vi "Unlock Data.vi"(8 "error in (no error)":errorcluster, 9 "Datum Type":variant, 10 "Datum Name":string, 11 "IModel in":refnum<class "IModel.lvclass">) -> (0 "error out":errorcluster, 3 "IModel out":refnum<class "IModel.lvclass">)   [LabVIEW 2015, in "IModel.lvlib" / "IModel.lvclass"]
doc: "Publish a datum (value) to the mediator bus. Published data are observable by any actor with access to the mediated bus."
uses:
  IModel.lvclass
  <vilib>/ActorFramework/Actor/Actor.lvclass/Actor.ctl
  <vilib>/ActorFramework/Message Enqueuer/Message Enqueuer.lvclass/Message Enqueuer.ctl
  IModel.lvclass/IModel.ctl
  AbstractMessages/PreAddressedMsg/PreAddressedMsg.lvclass/PreAddressedMsg.ctl
  IMediator/IMediator Messages/Unlock Publication Msg/Unlock Publication Msg.lvclass/Unlock Publication Msg.ctl
  <vilib>/ActorFramework/Actor/Read Self Enqueuer.vi
  <vilib>/ActorFramework/Message Enqueuer/Enqueue.vi
  AbstractMessages/PreAddressedMsg/Read Return Address.vi
  <vilib>/ActorFramework/Message Enqueuer/Init from Existing Queue.vi
  <vilib>/ActorFramework/Message Priority Queue/Priority Enqueue.vi
  <vilib>/ActorFramework/Message Enqueuer/Message Enqueuer.lvclass
  IObserver/IObserver/IObserver.lvclass
  IMediator/IMediator Messages/Unlock Publication Msg/Unlock Publication Msg.lvclass
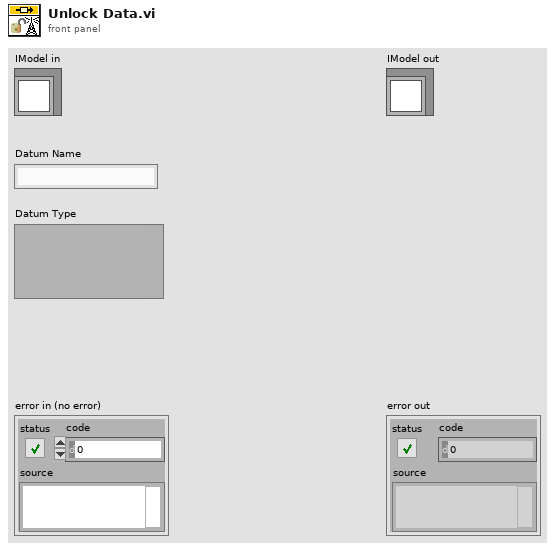
[diagram p1: front panel]
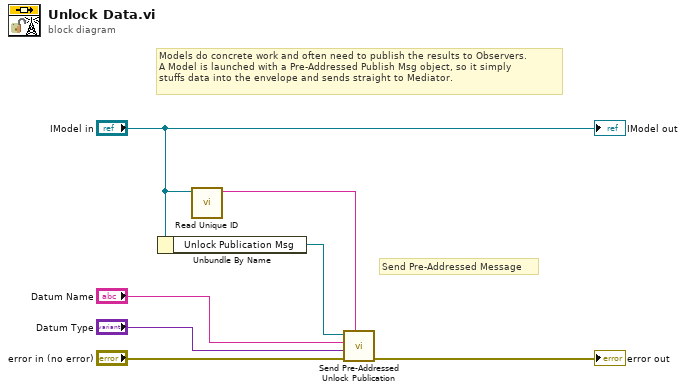
[diagram p0: block diagram]
diagram:
  # "Models do concrete work and often need to publish the results to Observers.\nA Model is launched with a Pre-Addressed Publish Msg object, so it simply\nstuffs data into the envelope and sends straight to Mediator."
  # "Send Pre-Addressed Message"
  n1 = Unbundle By Name("IModel in") -> ("Unlock Publication Msg"=w7:refnum<class "Unlock Publication Msg.lvclass">)
  n2 = call "Read Unique ID.vi"("IObserver In"="IModel in") -> ("Unique ID"=w3:string)  [unwired: 10 in]
  n3 = call "Send Pre-Addressed Unlock Publication.vi"("Publisher ID"=w3, "error in (no error)"="error in (no error)", "Data to Publish"="Datum Type", "Datum Name"="Datum Name", "Unlock Publication Msg"=w7) -> ("error out"=→"error out":errorcluster)  [unwired: 6 in]
  "IModel out" <- "IModel in"
